vi "总磷单步调试对话框.vi"() -> ()   [LabVIEW 2016, in "斯坦道总磷.lvlib"]
panel:
  in  "停止":bool
  out "温度2":sgl
  out "温度1":sgl
  out "ADC":sgl
  out "F3":sgl format="%#.6f"
  out "F2":sgl format="%#.6f"
  out "F1":sgl format="%#.6f"
  out "F0":sgl format="%#.6f"
  in  "退出":bool
  in  "启动":bool
  in  "总磷氨氮调试":u16[](xcontrol)
  # "单步调试界面"
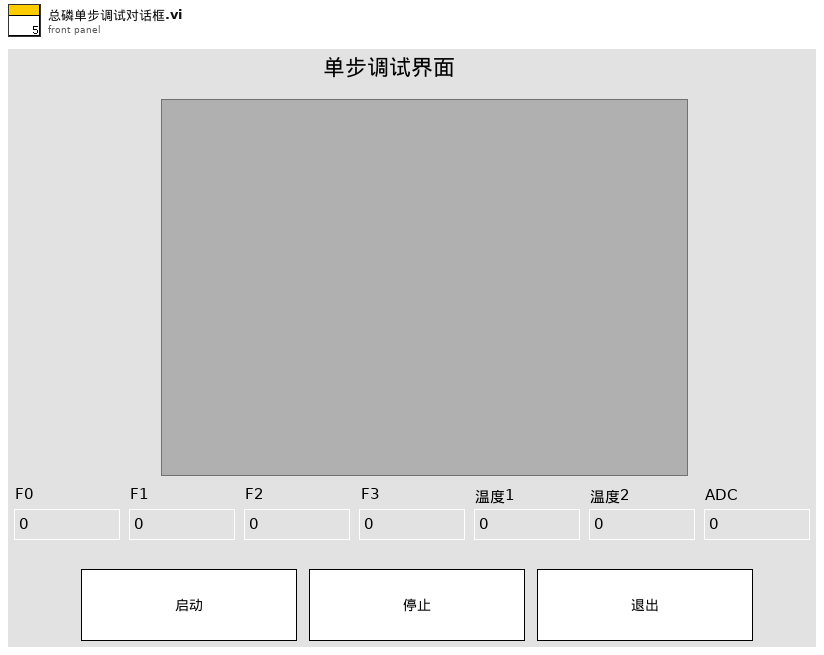
[diagram p1: front panel]
types:
  T1 = cluster{"V1":string, "V2":string, "V3":string, "V4":string, "V5":string, "V6":string, "V7":string, "V8":string, "V9":string, "V10":string, "V11":string, "V12":string, "V9-1":string, "V9-2":string}
  T2 = enum16{"自定义", "微站总磷总氮", "微站总磷氨氮", "微站氨氮", "固定站总磷", "固定站总氮", "固定站氨氮", "原位总磷总氮", "原位总磷氨氮", "原位总磷", "原位总氮", "原位氨氮", "原位3N1P"}
  T3 = cluster{"阀口名称自定义类型":enum16{"自定义", "微站总磷总氮", "微站总磷氨氮", "微站氨氮", "固定站总磷", "固定站总氮", "固定站氨氮", "原位总磷总氮", "原位总磷氨氮", "原位总磷", "原位总氮", "原位氨氮", "原位3N1P"}, "阀口自定义名称":cluster{"V1":string, "V2":string, "V3":string, "V4":string, "V5":string, "V6":string, "V7":string, "V8":string, "V9":string, "V10":string, "V11":string, "V12":string, "V9-1":string, "V9-2":string}}
  T4 = cluster{"系统时间":timestamp, "工作状态":enum16{"空闲", "水样测试", "标样核查", "零点核查", "跨度核查", "空白测试", "平行样测试", "加标回收", "空白校准", "标样校准", "初始化（清洗）"}, "测量模式":enum16{"待机", "连续模式", "周期模式", "定点模式", "受控模式", "手动模式"}, "告警代码":u16, "故障代码":u16, "日志代码":u16, "软件版本":u16, "F0":sgl, "F1":sgl, "F2":sgl, "F3":sgl, "T":sgl, "H":sgl, "id":u16, "flowid":u16, "量程":u16, "总磷控温温度1":sgl, "营养盐控温温度2":sgl, "ADC":sgl}
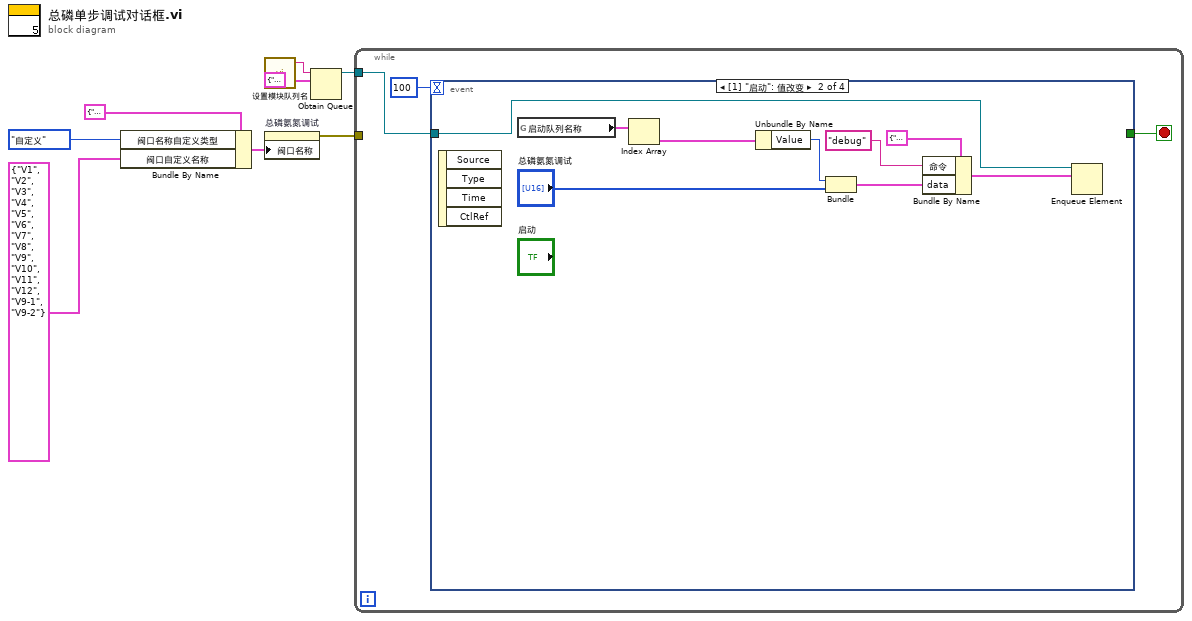
[diagram p0: block diagram]
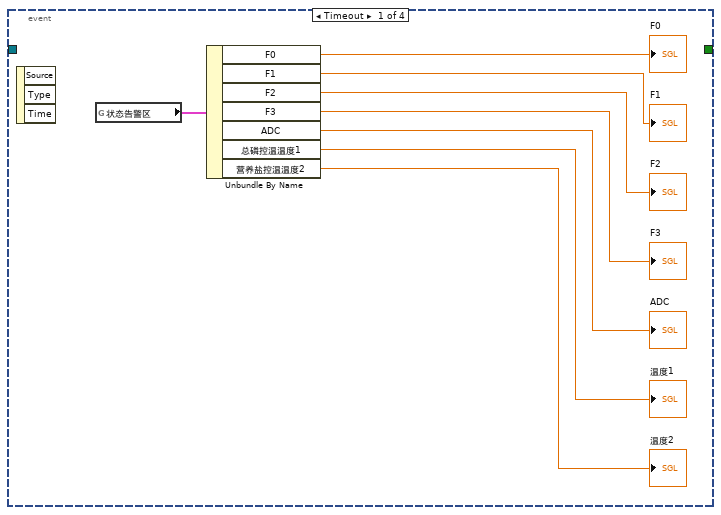
[diagram p2: hidden frame]
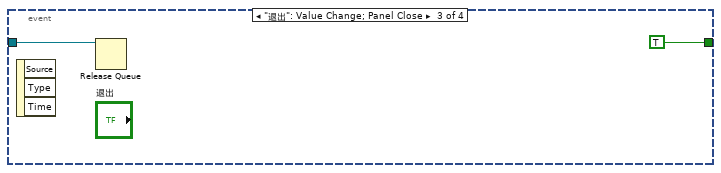
[diagram p3: hidden frame]
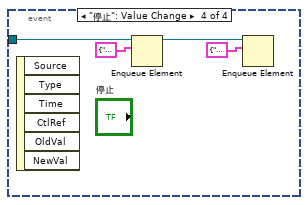
[diagram p4: hidden frame]
diagram:
  n1 = Bundle By Name(cluster=T3 {"阀口名称自定义类型"=enum."自定义", "阀口自定义名称"={"V1"="", "V2"="", "V3"="", "V4"="", "V5"="", "V6"="", "V7"="", "V8"="", "V9"="", "V10"="", "V11"="", "V12"="", "V9-1"="", "V9-2"=""}} ("阀口名称"), "阀口名称自定义类型"=T2."自定义", "阀口自定义名称"=T1 {"V1"="V1", "V2"="V2", "V3"="V3", "V4"="V4", "V5"="V5", "V6"="V6", "V7"="V7", "V8"="V8", "V9"="V9", "V10"="V10", "V11"="V11", "V12"="V12", "V9-1"="V9-1", "V9-2"="V9-2"}) -> (w5:T3)
  n2 = call "设置模块队列名.vi"() -> ("Msg"=w2:string)  [unwired: 5 in]
  n3 = property on="总磷氨氮调试" class="调试控件V3 (严格)"("阀口名称"=w5) -> (error out=w6:errorcluster)  [unwired: 2 in, 1 out]
  n4 = Obtain Queue(name (unnamed)=w2, element data type=cluster{"命令":string, "data":variant} {"命令"="", "data"=variant}) -> (queue out=w7:refnum<queue>)  [unwired: 3 in, 2 out]
  n5 = while {
    tunnel: w7 -> [w11]
    tunnel: w6 -> [_]
    stop <- w10 stop-if-true
    n6 = event shown="[1] \"启动\": 值改变" {
      selector: _ -> [_ _ _ _]
      dyn-events: _ -> [_ _ _ _]
      timeout: 100 -> [_ _ _ _]
      tunnel: w11 -> [_ w24 w29 w31]
      tunnel: [_ _ TRUE _] -> w10
      event Timeout {
        n7 = event-data() -> ()  [unwired: 1 in, 3 out]
        n8 = global read "VAR总磷总氮全局变量.vi" "状态告警区"() -> (w12:T4)
        n9 = Unbundle By Name(w12) -> ("F0"=→"F0":sgl, "F1"=→"F1":sgl, "F2"=→"F2":sgl, "F3"=→"F3":sgl, "ADC"=→"ADC":sgl, "总磷控温温度1"=→"温度1":sgl, "营养盐控温温度2"=→"温度2":sgl)
      }
      event "启动": Value Change {
        n10 = event-data() -> ()  [unwired: 1 in, 4 out]
        n11 = global read "VAR总磷总氮全局变量.vi" "启动队列名称"() -> (w22:cluster{"String":string, "Value":u16}[])
        n12 = Index Array(array=w22) -> (element=w21:cluster{"String":string, "Value":u16})  [unwired: 1 in]
        n13 = Unbundle By Name(w21) -> ("Value"=w20:u16)
        n14 = Bundle("Value"=w20, "总磷氨氮调试"="总磷氨氮调试") -> (w25:cluster{"Value":u16, "总磷氨氮调试":u16[]})  [unwired: 1 in]
        n15 = Bundle By Name(cluster=cluster{"命令":string, "data":variant} {"命令"="", "data"=variant} ("元素"), "命令"="debug", "data"=w25) -> (w26:cluster{"命令":string, "data":variant})
        n16 = Enqueue Element(queue=w24, element=w26) -> ()  [unwired: 2 in, 3 out]
      }
      event "退出": Value Change; Panel Close {
        n17 = event-data() -> ()  [unwired: 1 in, 3 out]
        n18 = Release Queue(queue=w29) -> ()  [unwired: 2 in, 3 out]
      }
      event "停止": Value Change {
        n19 = event-data() -> ()  [unwired: 1 in, 6 out]
        n20 = Enqueue Element(queue=w31, element=cluster{"命令":string, "data":variant} {"命令"="启动", "data"=variant(cluster{"站号":u16, "控制命令输出":u16[]} {"站号"=1, "控制命令输出"=[2816]})} ("元素")) -> (queue out=w32:refnum<queue>)  [unwired: 2 in, 2 out]
        n21 = Enqueue Element(queue=w32, element=cluster{"命令":string, "data":variant} {"命令"="启动", "data"=variant(cluster{"站号":u16, "控制命令输出":u16[]} {"站号"=2, "控制命令输出"=[2816]})} ("元素")) -> ()  [unwired: 2 in, 3 out]
      }
    }
  }
